vi "Really Simple Data Logger (RT).vi"() -> ()   [LabVIEW 2013]
uses:
  <vilib>/Utility/file.llb/Write To Spreadsheet File (string).vi
  <vilib>/FPGAPlugInAG/sbRIO-9626/niLvFpga_Open_sbRIO-9626.vi
  <vilib>/rvi/interface/common/dynamic/niFpgaDynamicAddResources.vi
  <vilib>/rvi/interface/common/niFpgaWaitOnOcc.vi
  <vilib>/Utility/error.llb/Error Cluster From Error Code.vi
  <vilib>/rvi/errors/niLvFpgaAdjustHostInterfaceError.vi
  <vilib>/rvi/interface/nirviOpenFPGA/nirviOpenFPGA.xnode
  FPGA Bitfiles/TIsbRIO_FPGATarget_ReallySimpleData_7aIvo7aPdC8.lvbitx
  FPGA/Really Simple Data Logger (FPGA).vi
  <vilib>/rvi/interface/nirviReadWriteControl/nirviReadWriteControl.xnode
  <vilib>/ptbypt/NI_PtbyPt.lvlib
  <vilib>/NI_Real-Time Target Support.lvlib
  NiFpgaLv.dll
  <vilib>/rvi/interface/Simulation/niFpgaSimulationCallBeginRW.vi
panel:
  out "Total (%)":dbl=7.457403564759815
  out "Log Data":bool
  in  "pb.Stop Profile":bool
  in  "pb.Run Profile":bool
  in  "Log Data Point":bool[](array[boolean])=[FALSE, FALSE, TRUE, FALSE, FALSE, FALSE, FALSE]
  in  "Sequencer":dbl[][](array[numeric])=[[1.0, 14.0], [2.0, 8.5], [2.0, 8.5], [5.0, 0.0]]
  out "Raw Cmd":dbl=2.1199
  out "Actual (V)":dbl=7.611040878295898 format="%.1f"
  in  "Offset":dbl
  in  "Scale":dbl=0.2494
  in  "PS Cmd (V)":dbl=8.5
  out "Actual":dbl[](array[numeric])=[7.611040878295898, 10.081106179809574, 0.16289023475646972, 9.2694348815918, 601.6718920742028, 301.8499590511331, 599.7986727725977] format="%.1f"
  in  "Offset":dbl[](array[numeric])=[0.0, -60.8, -60.7, -60.8, -256.333, -258.27, -258.96, 0.0, 0.0, 0.0, 0.0, 0.0, 0.0, 0.0, 0.0, 0.0]
  in  "Scale":dbl[](array[numeric])=[2.0, 24.038, 24.038, 24.038, 258.457, 258.27, 258.926, 0.0, 0.0, 0.0, 0.0, 0.0, 0.0, 0.0, 0.0, 0.0]
  out "Channel":string[](array[string])=["AI-0", "AI-1", "AI-2", "AI-3", "AI-4", "AI-5", "AI-6", "AI-7", "AI-8", "AI-9", "AI-10", "AI-11", "AI-12", "AI-13", "AI-14", "AI-15"]
  out "Description":string[](array[string])=["Power Supply (V)", "Pump 1 Current (A)", "Pump 2 Current (A)", "Pump 3 Current (A)", "Pump 1 Pressure (kPa)", "Pump 2 Pressure (kPa)", "Pump 3 Pressure (kPa)", "", "", "", "", "", "", "", "", ""]
  out "Raw Data (V)":dbl[](array[numeric])=[3.842355728149414, 2.9198684692382812, 2.530729293823242, 2.911235809326172, 3.3214778900146484, 2.171327590942383, 3.3138046264648438, 1.7748336791992188, -8.183547973632812, -4.07568359375, -2.3685226440429688, -1.4118232727050781, -0.8401050567626953, -0.4452095031738281, -0.1954822540283203, 0.0027637481689453125]
  # "Really Simple Data Logger v1.0"
  # "Time (sec)"
  # "PS Cmd (V)"
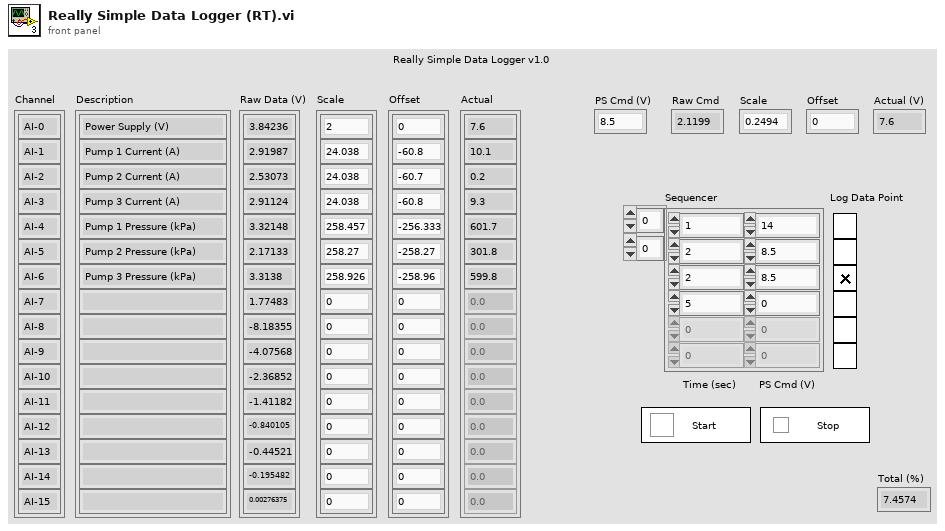
[diagram p1: front panel]
types:
  T1 = typedef "NI_Real-Time Target Support.lvlib/RT CPU Load.ctl" = cluster{"Total (%)":dbl, "Time Critical (%)":dbl, "Timed Structures (%)":dbl, "High (%)":dbl, "Above Normal (%)":dbl, "Normal (%)":dbl, "Background (%)":dbl, "Idle (%)":dbl, "ISR (%)":dbl}
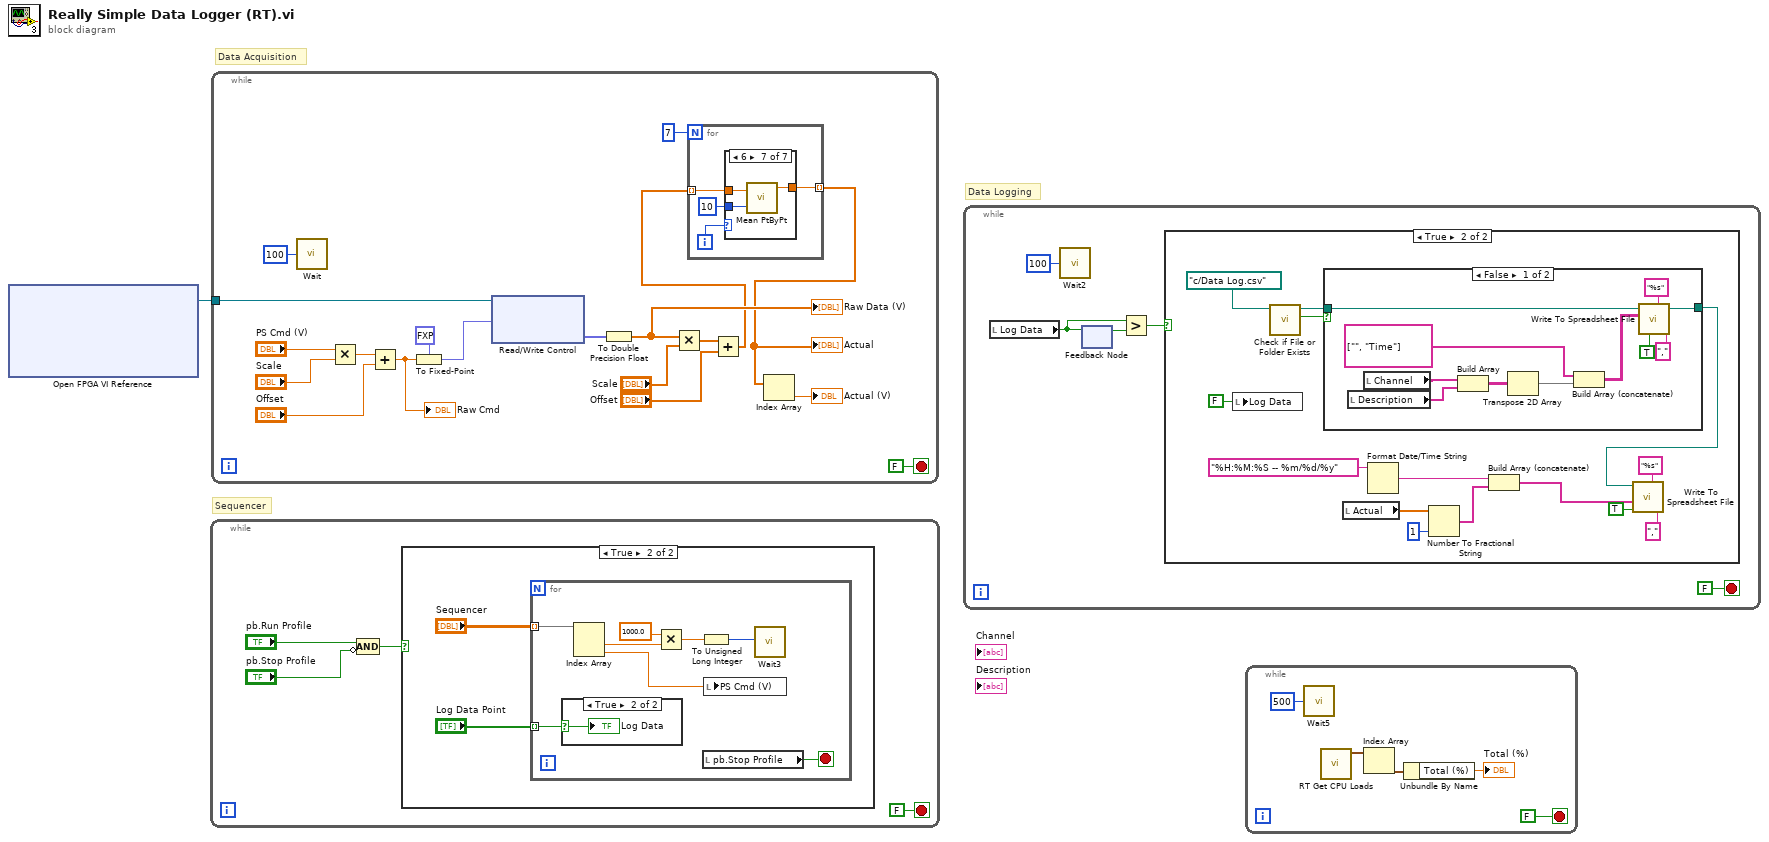
[diagram p0: block diagram]
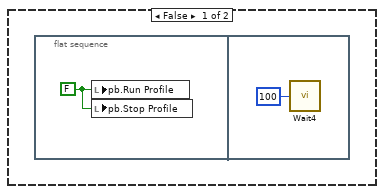
[diagram p4: hidden frame]
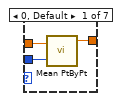
[diagram p6: hidden frame]
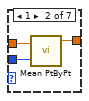
[diagram p7: hidden frame]
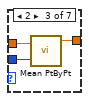
[diagram p8: hidden frame]
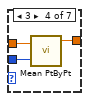
[diagram p9: hidden frame]
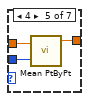
[diagram p10: hidden frame]
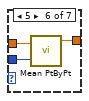
[diagram p11: hidden frame]
diagram:
  # "Data Logging"
  # "Sequencer"
  # "Data Acquisition"
  n1 = xnode "Open FPGA VI Reference"() -> ("FPGA VI Reference Out"=w1:refnum<k20>)  [unwired: 2 in, 1 out]
  n2 = while {
    stop <- FALSE stop-if-true
    n3 = Compound Arithmetic op=AND("pb.Run Profile", invert "pb.Stop Profile") -> (w3:bool)
    n4 = case shown="True" w3 {
      frame False {
        n5 = flat-sequence {
          frame #0 {
            w6 = FALSE ("pb.Run Profile")
            n6 = local write "pb.Run Profile"(w6) -> ()
            n7 = local write "pb.Stop Profile"(w6) -> ()
          }
          frame #1 {
            n8 = call "Wait4"("Count(mSec)"=u32 100) -> ()  [unwired: 1 out]
          }
        }
      }
      frame True {
        n9 = for {
          tunnel: "Sequencer" -> [w17] mode=indexing
          tunnel: "Log Data Point" -> [w10] mode=indexing
          stop <- w11 stop-if-true
          n10 = case shown="True" w10 {
            selector: w10 -> [_ w18]
            frame False {
            }
            frame True {
              "Log Data" <- w18
            }
          }
          n11 = Index Array(array=w17) -> (element #1=w16:dbl, element #2=w12:dbl)  [unwired: 2 in]
          n12 = Multiply(x=1000.0, y=w16) -> (x*y=w14:dbl)
          n13 = To Unsigned Long Integer(number=w14) -> (unsigned 32bit integer=w13:u32)
          n14 = local read "pb.Stop Profile"() -> (w11:bool)
          n15 = local write "PS Cmd (V)"(w12) -> ()
          n16 = call "Wait3"("Count(mSec)"=w13) -> ()  [unwired: 1 out]
        }
      }
    }
  }
  n17 = while {
    tunnel: w1 -> [w37]
    stop <- FALSE stop-if-true
    n18 = call "Wait"("Count(mSec)"=u32 100) -> ()  [unwired: 1 out]
    n19 = Multiply(x="PS Cmd (V)", y="Scale") -> (x*y=w34:dbl)
    n20 = Add(x=w34, y="Offset") -> (x+y=w24:dbl)
    "Raw Cmd" <- w24
    n21 = To Fixed-Point(fixed-point type=fxp<+/-,20,5> 0.0 ("AO0"), number=w24) -> (fixed-point=w31:fxp<+/-,20,5>)
    n22 = xnode "Read/Write Control"("FPGA VI Reference In"=w37, "AO0"=w31) -> ("Analog Inputs"=w30:fxp<+/-,24,5>[])  [unwired: 1 in, 2 out]
    n23 = To Double Precision Float(number=w30) -> (double precision float=w29:dbl[])
    "Raw Data (V)" <- w29
    n24 = Multiply(x=w29, y="Scale") -> (x*y=w27:dbl[])
    n25 = Add(x=w27, y="Offset") -> (x+y=w20:dbl[])
    n26 = for {
      N: 7 -> [_]
      tunnel: w20 -> [w40] mode=indexing
      tunnel: [w39] -> w19 mode=indexing
      i -> [w41]
      n27 = case shown="6" w41 {
        tunnel: w40 -> [w44 w47 w50 w53 w56 w59 w62]
        tunnel: [w43 w46 w49 w52 w55 w58 w61] -> w39
        tunnel: 10 ("sample length") -> [w42 w45 w48 w51 w54 w57 w60]
        frame 0, Default {
          n28 = call <vilib>:"Mean PtByPt.vi"("x"=w44, "sample length"=w42) -> ("mean"=w43:dbl)  [unwired: 2 in, 1 out]
        }
        frame 1 {
          n29 = call <vilib>:"Mean PtByPt.vi"("x"=w47, "sample length"=w45) -> ("mean"=w46:dbl)  [unwired: 2 in, 1 out]
        }
        frame 2 {
          n30 = call <vilib>:"Mean PtByPt.vi"("x"=w50, "sample length"=w48) -> ("mean"=w49:dbl)  [unwired: 2 in, 1 out]
        }
        frame 3 {
          n31 = call <vilib>:"Mean PtByPt.vi"("x"=w53, "sample length"=w51) -> ("mean"=w52:dbl)  [unwired: 2 in, 1 out]
        }
        frame 4 {
          n32 = call <vilib>:"Mean PtByPt.vi"("x"=w56, "sample length"=w54) -> ("mean"=w55:dbl)  [unwired: 2 in, 1 out]
        }
        frame 5 {
          n33 = call <vilib>:"Mean PtByPt.vi"("x"=w59, "sample length"=w57) -> ("mean"=w58:dbl)  [unwired: 2 in, 1 out]
        }
        frame 6 {
          n34 = call <vilib>:"Mean PtByPt.vi"("x"=w62, "sample length"=w60) -> ("mean"=w61:dbl)  [unwired: 2 in, 1 out]
        }
      }
    }
    "Actual" <- w19
    n35 = Index Array(array=w19) -> (element=→"Actual (V)":dbl)  [unwired: 1 in]
  }
  n36 = while {
    stop <- FALSE stop-if-true
    n37 = local read "Log Data"() -> (w66:bool)
    n38 = call "Wait2"("Count(mSec)"=u32 100) -> ()  [unwired: 1 out]
    n39 = feedback-in #1(w66) -> ()
    n40 = feedback #1() -> (w65:bool)  [unwired: 1 in]
    n41 = Greater?(x=w66, y=w65) -> (0:w64:bool)
    n42 = case shown="True" w64 {
      frame False {
      }
      frame True {
        n43 = local write "Log Data"(FALSE ("Log Data")) -> ()
        n44 = call <vilib>:"Check if File or Folder Exists.vi"("path"=path "c:/Data Log.csv") -> ("file or folder exists?"=w80:bool, "dup path"=w79:path)  [unwired: 8 in, 1 out]
        n45 = case shown="False" w80 {
          tunnel: w79 -> [w88 w93]
          tunnel: [w84 w93] -> w76
          frame False {
            n46 = local read "Description"() -> (w90:string[])
            n47 = local read "Channel"() -> (w89:string[])
            n48 = Build Array(w89, w90) -> (w91:string[][])
            n49 = Transpose 2D Array(2D array=w91) -> (transposed array=w82:string[][])
            n50 = Build Array (concatenate)(string[] ["", "Time"], w82) -> (w87:string[][])
            n51 = call-poly <vilib>:"Write To Spreadsheet File.vi"("delimiter (\\t)"="," ("delimiter (\\t)"), "transpose? (no:F)"=TRUE, "format (%s)"="%s", "2D data"=w87, "file path (dialog if empty)"=w88) -> ("new file path (Not A Path if cancelled)"=w84:path)  [unwired: 3 in]
          }
          frame True {
          }
        }
        n52 = local read "Actual"() -> (w73:dbl[])
        n53 = Format Date/Time String(time format string (%c)="%H:%M:%S -- %m/%d/%y") -> (date/time string=w71:string)  [unwired: 2 in]
        n54 = Number To Fractional String(number=w73, precision (6)=i16 1) -> (F-format string=w70:string[])  [unwired: 2 in]
        n55 = Build Array (concatenate)(w71, w70) -> (w69:string[])
        n56 = call-poly <vilib>:"Write To Spreadsheet File.vi"("delimiter (\\t)"="," ("delimiter (\\t)"), "format (%s)"="%s", "append to file? (new file:F)"=TRUE, "1D data"=w69, "file path (dialog if empty)"=w76) -> ()  [unwired: 3 in, 1 out]
      }
    }
  }
  n57 = while {
    stop <- FALSE stop-if-true
    n58 = call "Wait5"("Count(mSec)"=u32 500) -> ()  [unwired: 1 out]
    n59 = call <vilib>:"RT Get CPU Loads.vi"() -> ("CPU loads"=w98:T1[])  [unwired: 10 in, 1 out]
    n60 = Index Array(array=w98) -> (element=w97:T1)  [unwired: 1 in]
    n61 = Unbundle By Name(w97) -> ("Total (%)"=→"Total (%)":dbl)
  }
